vi "Acquire_CCD_data.vi"(6 "readout_stride (bytes)":i32, 7 "frame size (bytes)":i32, 8 "error in":errorcluster, 9 "readout_time_out (ms)":i32=4000, 10 "readout_count":i64=1, 11 "camera handle in":u64) -> (0 "error out":errorcluster, 1 "read_count * frames":u16[][](array[numeric]), 3 "camera handle out":u64, 4 "Errors_out":u32)   [LabVIEW 2014, in "PICam.lvlib"]
doc: "Picam_Acquire() performs a specified number of data readouts (specified by readout_count) and returns once the acquisition has been completed."
uses:
  PICam.lvlib
  Picam32.dll
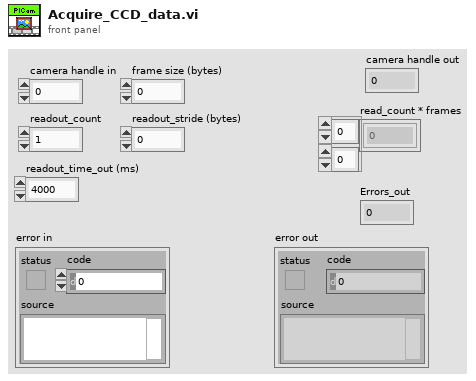
[diagram p1: front panel]
types:
  T1 = cluster{"initial_readout*":u64, "readout_count":i64}
  T2 = cluster{"initial_readout*":u32, "dummy filler":u32, "readout_count":i64}
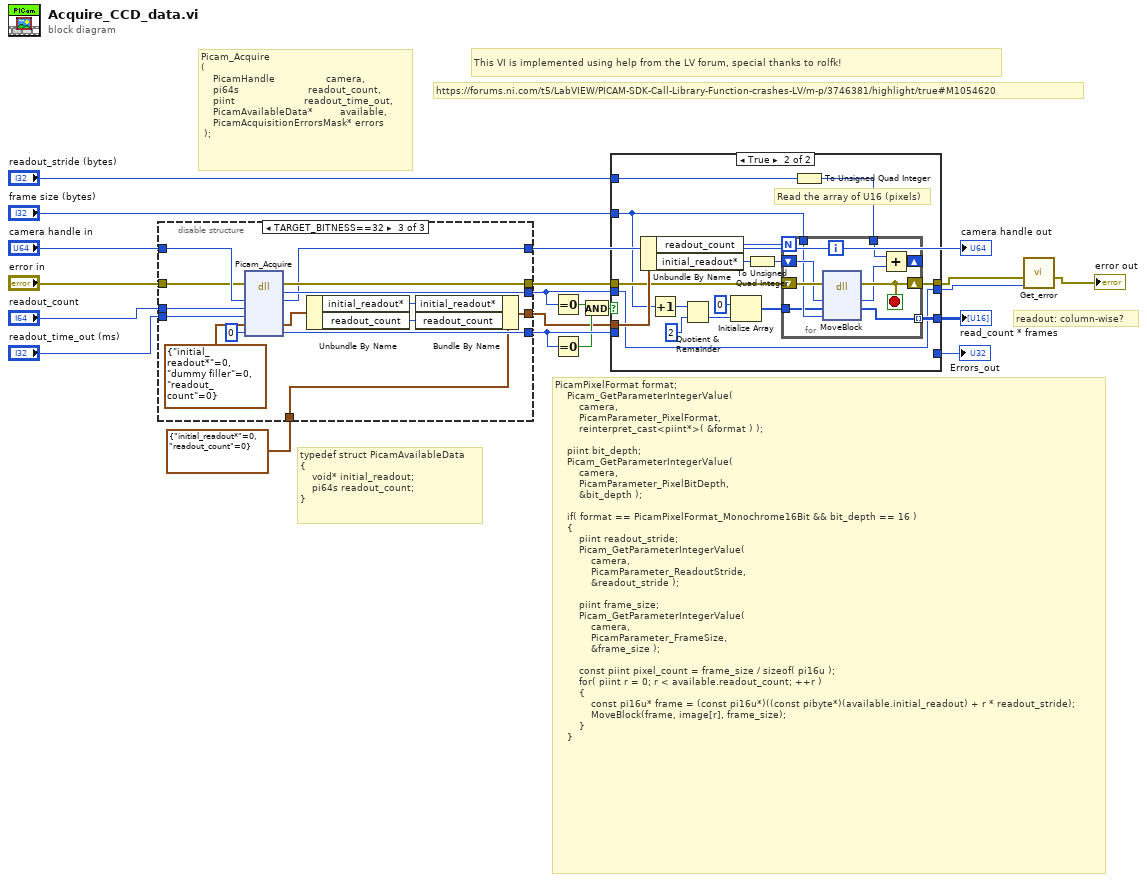
[diagram p0: block diagram]
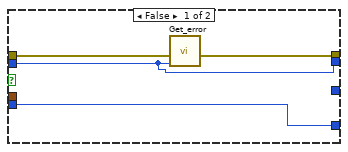
[diagram p2: hidden frame]
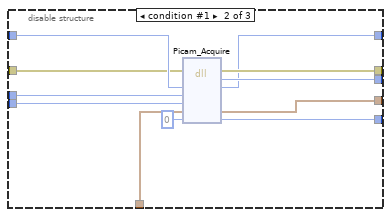
[diagram p4: hidden frame]
diagram:
  # "readout: column-wise?"
  # "https://forums.ni.com/t5/LabVIEW/PICAM-SDK-Call-Library-Function-crashes-LV/m-p/3746381/highlight/true#M1054620"
  # "This VI is implemented using help from the LV forum, special thanks to rolfk!"
  # "PicamPixelFormat format;\n    Picam_GetParameterIntegerValue(\n        camera,\n        PicamParameter_PixelFormat,\n        reinterpret_cast<piint*>( &format ) );\n\n    piint bit_depth;\n    Picam_GetParameterIntegerValue(\n        camera,\n        PicamParameter_PixelBitDepth,\n        &bit_depth );\n\n    if( format == PicamPixelFormat_Monochrome16Bit && bit_depth == 16 )\n    {\n        piint readout_stride;\n        Picam_GetParameterIntegerValue(\n            camera,\n            PicamParameter_ReadoutStride,\n            &readout_stride );\n\n        piint frame_size;\n        Picam_GetParameterIntegerValue(\n            camera,\n            PicamParameter_FrameSize,\n            &frame_size );\n\n        const piint pixel_count = frame_size / sizeof( pi16u );\n        for( piint r = 0; r < available.readout_count; ++r )\n        {\n            const pi16u* frame = (const pi16u*)((const pibyte*)(available.initial_readout) + r * readout_stride);\n            MoveBlock(frame, image[r], frame_size);\n        }\n    }"
  # "Picam_Acquire\n(\n    PicamHandle                 camera,\n    pi64s                       readout_count,\n    piint                       readout_time_out,\n    PicamAvailableData*         available,\n    PicamAcquisitionErrorsMask* errors\n );"
  # "typedef struct PicamAvailableData\n{\n    void* initial_readout;\n    pi64s readout_count;\n}"
  n1 = disable-structure shown="TARGET_BITNESS==32" {
    disable-tunnel: [w21 w33 w48] -> w20
    disable-tunnel: [_ w32 w47] -> w13
    disable-tunnel: "camera handle in" -> [w22 w31 w46]
    disable-tunnel: "error in" -> [w21 w30 w45]
    disable-tunnel: [w22 w29 w44] -> w17
    disable-tunnel: "readout_count" -> [_ w28 w43]
    disable-tunnel: "readout_time_out (ms)" -> [_ w27 w42]
    disable-tunnel: [_ w26 w41] -> w14
    disable-tunnel: [_ w23 w36] -> w10
    disable-tunnel: T1 {"initial_readout*"=0, "readout_count"=0} -> [_ w25 w37]
    frame condition #0 {
    }
    frame condition #1 {
      n2 = dll-call lib="Picam32.dll" fn="Picam_Acquire"(error in=w30, "camera"=w31, "readout_count"=w28, "readout_time_out"=w27, "PicamAvailableData"=w25, "Errors_out"=u32 0) -> (error out=w33:errorcluster, "return type"=w32:i32, "camera"=w29:u64, "PicamAvailableData"=w23:T1, "Errors_out"=w26:u32)  [unwired: 4 in, 1 out]
    }
    frame condition #2 (active) {
      n3 = dll-call lib="Picam32.dll" fn="Picam_Acquire"(error in=w45, "camera"=w46, "readout_count"=w43, "readout_time_out"=w42, "PicamAvailableData"=T2 {"initial_readout*"=0, "dummy filler"=0, "readout_count"=0}, "Errors_out"=u32 0) -> (error out=w48:errorcluster, "return type"=w47:i32, "camera"=w44:u64, "PicamAvailableData"=w38:T2, "Errors_out"=w41:u32)  [unwired: 4 in, 1 out]
      n4 = Unbundle By Name(w38) -> ("initial_readout*"=w35:u32, "readout_count"=w34:i64)
      n5 = Bundle By Name(cluster=w37, "initial_readout*"=w35, "readout_count"=w34) -> (w36:T1)
    }
  }
  "camera handle out" <- w17
  n6 = Equal To 0?(x=w13) -> (x = 0?=w12:bool)
  n7 = Equal To 0?(x=w14) -> (x = 0?=w11:bool)
  n8 = And(x=w12, y=w11) -> (x .and. y?=w9:bool)
  n9 = case shown="True" w9 {
    tunnel: w20 -> [w52 w67]
    tunnel: w13 -> [w49 w53]
    tunnel: w14 -> [w50 _]
    tunnel: w10 -> [_ w68]
    tunnel: "readout_stride (bytes)" -> [_ w64]
    tunnel: "frame size (bytes)" -> [_ w58]
    tunnel: [_ w56] -> w6
    tunnel: [w51 w55] -> w3
    tunnel: [w50 _] -> w5
    tunnel: [w49 w53] -> w1
    frame False {
      n10 = call "Get_error.vi"("PICam_Error"=w49, "error in (no error)"=w52) -> ("error out"=w51:errorcluster)  [unwired: 9 in]
    }
    frame True {
      # "Read the array of U16 (pixels)"
      n11 = Unbundle By Name(w68) -> ("readout_count"=w66:i64, "initial_readout*"=w65:u64)
      n12 = Increment(x=w58) -> (x+1=w61:i32)
      n13 = Quotient & Remainder(x=w61, y=2) -> (floor(x/y)=w59:i32)  [unwired: 1 out]
      n14 = Initialize Array(u16 0 ("element"), w59) -> (w57:u16[])
      n15 = To Unsigned Quad Integer(1:w65) -> (0:w54:u64)
      n16 = To Unsigned Quad Integer(1:w64) -> (0:w63:u64)
      n17 = for {
        N: w66 -> [_]
        shift-right: [w76] -> w55
        shift-left: w67 -> [w77]
        shift-right: [w74] -> _
        shift-left: w54 -> [w75]
        tunnel: w63 -> [w69]
        tunnel: w58 -> [w73]
        tunnel: w57 -> [w72]
        tunnel: [w71] -> w56 mode=indexing
        stop <- w76 stop-if-true
        n18 = dll-call lib="LabVIEW" fn="MoveBlock"(error in=w77, "src"=w75, "tgt"=w72, "size"=w73) -> (error out=w76:errorcluster, "src"=w70:u64, "tgt"=w71:u16[])  [unwired: 4 in, 1 out]
        n19 = Add(x=w69, y=w70) -> (x+y=w74:u64)
      }
    }
  }
  "Errors_out" <- w5
  "read_count * frames" <- w6
  n20 = call "Get_error.vi"("PICam_Error"=w1, "error in (no error)"=w3) -> ("error out"=→"error out":errorcluster)  [unwired: 9 in]
